vi "FRCts20_EspEngine_Event.vi"(8 "error in (no error)":errorcluster, 10 "Event":T1, 11 "httpRequestID":u32) -> (0 "error out":errorcluster, 3 "httpRequestID out":u32)   [LabVIEW 2014, in "FRCts20_EspEngine.lvlib"]
uses:
  FRCts20_EspEngine.lvlib
  TypeDefs/FRCts20_EspEngine_Event.ctl
  Web Methods/source/VI Source/Web Method Public Interface/FRCts20_WebMethods_ctl_singleEvent.ctl
  Web Methods/source/VI Source/Web Method Public Interface/FRCts20_WebMethods_ctl_teamIdentifier.ctl
  <vilib>/wsapi/subVIs/Set String ESP Variable.vi
  <vilib>/wsapi/subVIs/Set Integer ESP Variable.vi
  <vilib>/wsapi/subVIs/Set Boolean ESP Variable.vi
  <vilib>/wsapi/NI_WebServices.lvlib
  Web Methods/source/VI Source/FRCts20_WebMethods.lvlib
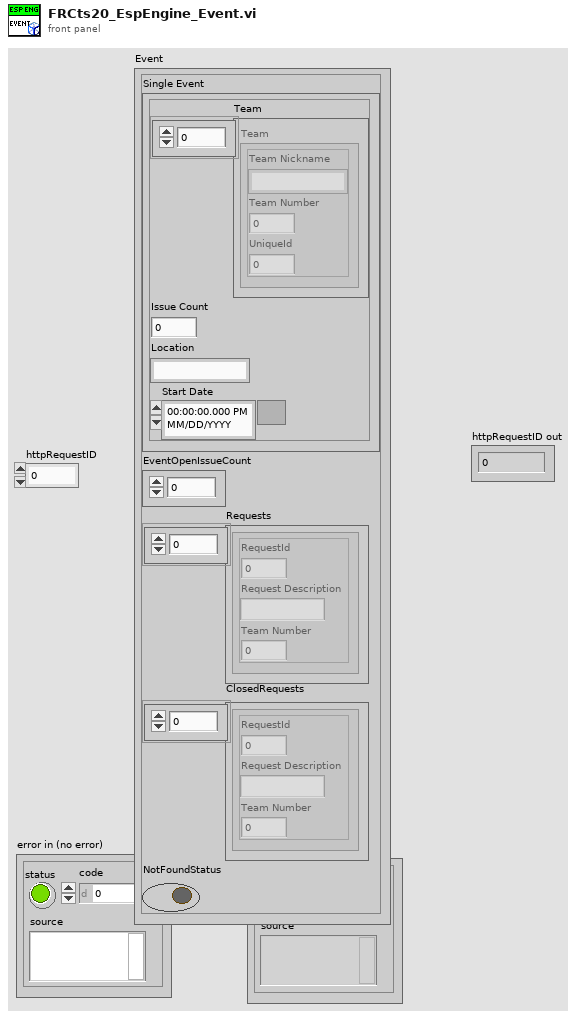
[diagram p1: front panel]
types:
  T1 = typedef "FRCts20_EspEngine.lvlib/FRCts20_EspEngine_Event.ctl" = cluster{"Single Event":T2, "EventOpenIssueCount":i16, "Requests":cluster{"RequestId":i32, "Request Description":string, "Team Number":i32}[], "ClosedRequests":cluster{"RequestId":i32, "Request Description":string, "Team Number":i32}[], "NotFoundStatus":bool}
  T2 = typedef "FRCts20_WebMethods.lvlib/FRCts20_WebMethods_ctl_singleEvent.ctl" = cluster{"Team":T3[], "Issue Count":i32, "Location":string, "Start Date ":timestamp}
  T3 = typedef "FRCts20_WebMethods.lvlib/FRCts20_WebMethods_ctl_teamIdentifier.ctl" = cluster{"Team Nickname":string, "Team Number ":u32, "UniqueId":u32}
  T4 = cluster{"RequestId":i32, "Request Description":string, "Team Number":i32}[]
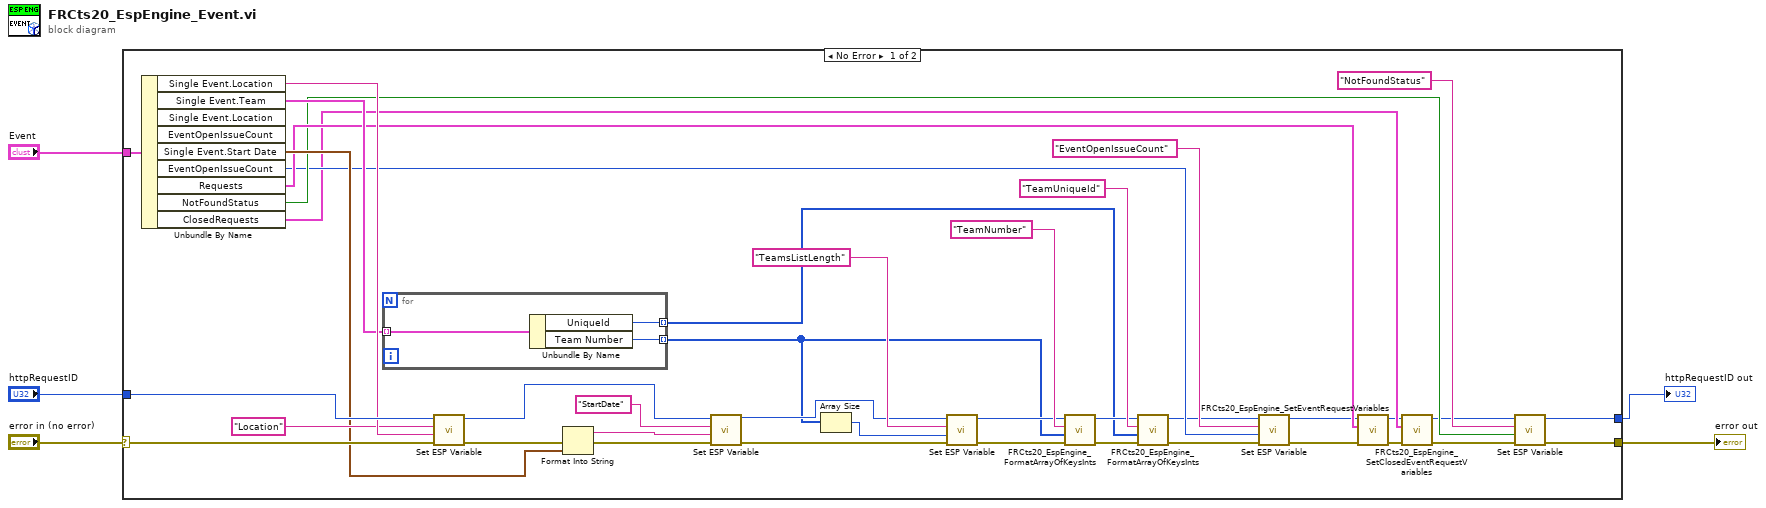
[diagram p0: block diagram]
diagram:
  n1 = case shown="No Error" "error in (no error)" {
    selector: "error in (no error)" -> [w40 w49]
    tunnel: [w20 w49] -> w5
    tunnel: "httpRequestID" -> [w45 _]
    tunnel: "Event" -> [w44 _]
    tunnel: [w19 _] -> w1
    frame No Error {
      n2 = Unbundle By Name(w44) -> ("Single Event.Location"=w43:string, "Single Event.Team"=w34:T3[], "Single Event.Start Date"=w32:timestamp, "EventOpenIssueCount"=w13:i16, "Requests"=w22:T4, "NotFoundStatus"=w18:bool, "ClosedRequests"=w10:T4)  [unwired: 2 out]
      n3 = for {
        tunnel: w34 -> [w48] mode=indexing
        tunnel: [w47] -> w24 mode=indexing
        tunnel: [w46] -> w17 mode=indexing
        n4 = Unbundle By Name(w48) -> ("UniqueId"=w47:u32, "Team Number"=w46:u32)
      }
      n5 = call-poly <vilib>:"Set ESP Variable.vi"("error in (no error)"=w40, "value"=w43, "key"="Location", "httpRequestID"=w45) -> ("error out"=w30:errorcluster, "httpRequestID out"=w38:u32)  [unwired: 6 in]
      n6 = Format Into String(error in=w30, w32) -> (resulting string=w31:string, error out=w29:errorcluster)  [unwired: 2 in]
      n7 = call-poly <vilib>:"Set ESP Variable.vi"("error in (no error)"=w29, "value"=w31, "key"="StartDate", "httpRequestID"=w38) -> ("error out"=w33:errorcluster, "httpRequestID out"=w37:u32)  [unwired: 6 in]
      n8 = Array Size(array=w17) -> (size(s)=w23:i32)
      n9 = call-poly <vilib>:"Set ESP Variable.vi"("error in (no error)"=w33, "value"=w23, "key"="TeamsListLength", "httpRequestID"=w37) -> ("error out"=w36:errorcluster, "httpRequestID out"=w26:u32)  [unwired: 6 in]
      n10 = call "FRCts20_EspEngine_FormatArrayOfKeysInts.vi"("error IO"=w36, "Values"=w17, "KeyBaseName"="TeamNumber", "httpRequestID"=w26) -> ("error IO"=w27:errorcluster, "httpRequestID out"=w25:u32)  [unwired: 6 in]
      n11 = call "FRCts20_EspEngine_FormatArrayOfKeysInts.vi"("error IO"=w27, "Values"=w24, "KeyBaseName"="TeamUniqueId", "httpRequestID"=w25) -> ("error IO"=w15:errorcluster, "httpRequestID out"=w8:u32)  [unwired: 6 in]
      n12 = call-poly <vilib>:"Set ESP Variable.vi"("error in (no error)"=w15, "value"=w13, "key"="EventOpenIssueCount", "httpRequestID"=w8) -> ("error out"=w14:errorcluster, "httpRequestID out"=w9:u32)  [unwired: 6 in]
      n13 = call "FRCts20_EspEngine_SetEventRequestVariables.vi"("error in (no error)"=w14, "Requests"=w22, "httpRequestID in"=w9) -> ("error out"=w12:errorcluster, "httpRequestID out"=w7:u32)  [unwired: 7 in]
      n14 = call "FRCts20_EspEngine_SetClosedEventRequestVariables.vi"("error in (no error)"=w12, "ClosedRequests"=w10, "httpRequestID in"=w7) -> ("error out"=w11:errorcluster, "httpRequestID out"=w6:u32)  [unwired: 7 in]
      n15 = call-poly <vilib>:"Set ESP Variable.vi"("error in (no error)"=w11, "value"=w18, "key"="NotFoundStatus", "httpRequestID"=w6) -> ("error out"=w20:errorcluster, "httpRequestID out"=w19:u32)  [unwired: 6 in]
    }
    frame Error {
    }
  }
  "error out" <- w5
  "httpRequestID out" <- w1
